vi "Get BMS into load mode.vi"(7 "timeout in ms (-1)":i32=-1, 8 "error in":errorcluster, 11 "CAN Session In":T1) -> (0 "error out":errorcluster, 2 "Error":bool, 3 "CAN Session Out":T1)   [LabVIEW 2016]
uses:
  Program Files (x86)/National Instruments/LabVIEW 2016/examples/robotics/EPOS2 CANOpen Driver/Low Level VIs/Typedefs/CAN Refnum.ctl
  Program Files (x86)/National Instruments/LabVIEW 2016/examples/robotics/EPOS2 CANOpen Driver/Low Level VIs/Typedefs/CAN Session Pointer.ctl
  Program Files (x86)/National Instruments/LabVIEW 2016/examples/robotics/EPOS2 CANOpen Driver/Low Level VIs/Typedefs/CAN Communication References.ctl
  Program Files (x86)/National Instruments/LabVIEW 2016/examples/robotics/EPOS2 CANOpen Driver/Low Level VIs/Typedefs/kill process notifier array.ctl
  Program Files (x86)/National Instruments/LabVIEW 2016/examples/robotics/EPOS2 CANOpen Driver/Low Level VIs/Typedefs/Write Queue.ctl
  Program Files (x86)/National Instruments/LabVIEW 2016/examples/robotics/EPOS2 CANOpen Driver/Low Level VIs/Typedefs/FPGA CAN Frame Cluster.ctl
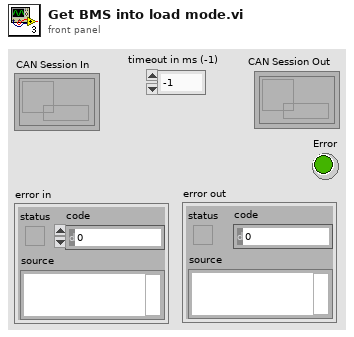
[diagram p1: front panel]
types:
  T1 = typedef "CAN Refnum.ctl" = refnum<k1>
  T2 = typedef "Stage Request Status.ctl" = cluster{"precharge done":bool, "staging ack":bool, "active request":bool}
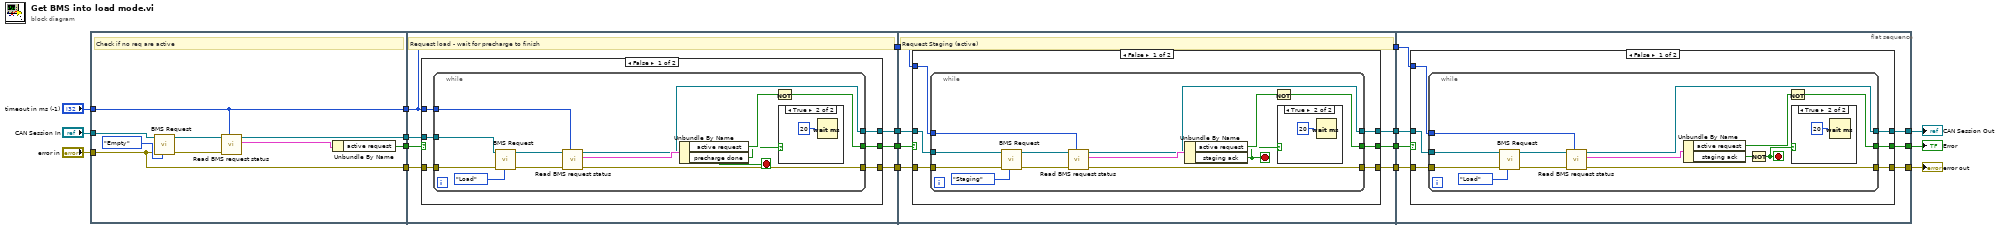
[diagram p0: block diagram]
diagram:
  n1 = flat-sequence {
    tunnel: "CAN Session In" -> [w21]
    tunnel: "error in" -> [w23]
    tunnel: "timeout in ms (-1)" -> [w19]
    tunnel: [w19] -> w15
    tunnel: [w20] -> w14
    tunnel: [w23] -> w13
    tunnel: [w22] -> w12
    tunnel: w15 -> [w28]
    tunnel: [w28] -> w11
    tunnel: w14 -> [w32]
    tunnel: w13 -> [w30]
    tunnel: w12 -> [w34]
    tunnel: [w31] -> w10
    tunnel: [w29] -> w9
    tunnel: [w33] -> w8
    tunnel: w11 -> [w57]
    tunnel: w10 -> [w63]
    tunnel: w9 -> [w62]
    tunnel: w8 -> [w61]
    tunnel: [w60] -> w7
    tunnel: [w59] -> w6
    tunnel: [w58] -> w5
    tunnel: [w57] -> w4
    tunnel: w7 -> [w92]
    tunnel: w6 -> [w89]
    tunnel: w5 -> [w90]
    tunnel: w4 -> [w91]
    tunnel: [w88] -> w3
    tunnel: [w87] -> w2
    tunnel: [w86] -> w1
    frame #0 {
      # "Check if no req are active"
      n2 = call "BMS Request.vi"("Request"=enum16{"Empty", "Load", "Staging"}."Empty", "error in"=w23, "CAN Session In"=w21) -> ("error out"=w25:errorcluster, "CAN Session Out"=w24:T1)  [unwired: 7 in]
      n3 = call "Read BMS request status.vi"("timeout in ms (-1)"=w19, "error in"=w25, "CAN Session In"=w24) -> ("Stage Request Status"=w27:T2, "CAN Session Out"=w20:T1)  [unwired: 6 in, 1 out]
      n4 = Unbundle By Name(w27) -> ("active request"=w22:bool)
    }
    frame #1 {
      # "Request load - wait for precharge to finish"
      n5 = case shown="False" w34 {
        selector: w34 -> [_ w56]
        tunnel: w32 -> [w40 w54]
        tunnel: w30 -> [w39 w55]
        tunnel: [w38 w56] -> w33
        tunnel: [w37 w54] -> w31
        tunnel: [w36 w55] -> w29
        tunnel: w28 -> [w35 _]
        frame False {
          n6 = while {
            tunnel: w40 -> [w48]
            tunnel: w39 -> [w46]
            tunnel: [w44] -> w38
            tunnel: [w43] -> w37
            tunnel: [w42] -> w36
            tunnel: w35 -> [w41]
            stop <- w45 stop-if-true
            n7 = call "BMS Request.vi"("Request"=enum16{"Empty", "Load", "Staging"}."Load", "error in"=w46, "CAN Session In"=w48) -> ("error out"=w52:errorcluster, "CAN Session Out"=w47:T1)  [unwired: 7 in]
            n8 = call "Read BMS request status.vi"("timeout in ms (-1)"=w41, "error in"=w52, "CAN Session In"=w47) -> ("error out"=w42:errorcluster, "Stage Request Status"=w50:T2, "CAN Session Out"=w43:T1)  [unwired: 6 in]
            n9 = Unbundle By Name(w50) -> ("active request"=w49:bool, "precharge done"=w45:bool)
            n10 = Not(x=w49) -> (.not. x?=w44:bool)
            n11 = case shown="True" w45 {
              frame False {
              }
              frame True {
                n12 = Wait (ms)(milliseconds to wait=u32 20) -> ()  [unwired: 1 out]
              }
            }
          }
        }
        frame True {
        }
      }
    }
    frame #2 {
      # "Request Staging (active)"
      n13 = case shown="False" w61 {
        selector: w61 -> [_ w85]
        tunnel: w63 -> [w69 w84]
        tunnel: w62 -> [w68 w83]
        tunnel: [w67 w85] -> w60
        tunnel: [w66 w83] -> w59
        tunnel: [w65 w84] -> w58
        tunnel: w57 -> [w64 _]
        frame False {
          n14 = while {
            tunnel: w69 -> [w77]
            tunnel: w68 -> [w76]
            tunnel: [w73] -> w67
            tunnel: [w72] -> w66
            tunnel: [w71] -> w65
            tunnel: w64 -> [w70]
            stop <- w74 stop-if-true
            n15 = call "BMS Request.vi"("Request"=enum16{"Empty", "Load", "Staging"}."Staging", "error in"=w76, "CAN Session In"=w77) -> ("error out"=w81:errorcluster, "CAN Session Out"=w75:T1)  [unwired: 7 in]
            n16 = call "Read BMS request status.vi"("timeout in ms (-1)"=w70, "error in"=w81, "CAN Session In"=w75) -> ("error out"=w72:errorcluster, "Stage Request Status"=w79:T2, "CAN Session Out"=w71:T1)  [unwired: 6 in]
            n17 = Unbundle By Name(w79) -> ("active request"=w78:bool, "staging ack"=w74:bool)
            n18 = Not(x=w78) -> (.not. x?=w73:bool)
            n19 = case shown="True" w74 {
              frame False {
              }
              frame True {
                n20 = Wait (ms)(milliseconds to wait=u32 20) -> ()  [unwired: 1 out]
              }
            }
          }
        }
        frame True {
        }
      }
    }
    frame #3 {
      n21 = case shown="False" w92 {
        selector: w92 -> [_ w115]
        tunnel: [w98 w115] -> w88
        tunnel: [w97 w113] -> w86
        tunnel: [w96 w114] -> w87
        tunnel: w91 -> [w95 _]
        tunnel: w90 -> [w94 w114]
        tunnel: w89 -> [w93 w113]
        frame False {
          n22 = while {
            tunnel: [w106] -> w98
            tunnel: [w105] -> w97
            tunnel: [w104] -> w96
            tunnel: w95 -> [w103]
            tunnel: w94 -> [w102]
            tunnel: w93 -> [w101]
            stop <- w99 stop-if-true
            n23 = call "BMS Request.vi"("Request"=enum16{"Empty", "Load", "Staging"}."Load", "error in"=w101, "CAN Session In"=w102) -> ("error out"=w111:errorcluster, "CAN Session Out"=w107:T1)  [unwired: 7 in]
            n24 = call "Read BMS request status.vi"("timeout in ms (-1)"=w103, "error in"=w111, "CAN Session In"=w107) -> ("error out"=w105:errorcluster, "Stage Request Status"=w109:T2, "CAN Session Out"=w104:T1)  [unwired: 6 in]
            n25 = Unbundle By Name(w109) -> ("active request"=w108:bool, "staging ack"=w100:bool)
            n26 = Not(x=w100) -> (.not. x?=w99:bool)
            n27 = Not(x=w108) -> (.not. x?=w106:bool)
            n28 = case shown="True" w99 {
              frame False {
              }
              frame True {
                n29 = Wait (ms)(milliseconds to wait=u32 20) -> ()  [unwired: 1 out]
              }
            }
          }
        }
        frame True {
        }
      }
    }
  }
  "Error" <- w3
  "CAN Session Out" <- w2
  "error out" <- w1
